vi "pane.vi"() -> ()   [LabVIEW 2015]
uses:
  <vilib>/Utility/miscctls.llb/LVPointTypeDef.ctl
panel:
  in  "Home":bool
  in  "User":bool
  in  "Devices":bool
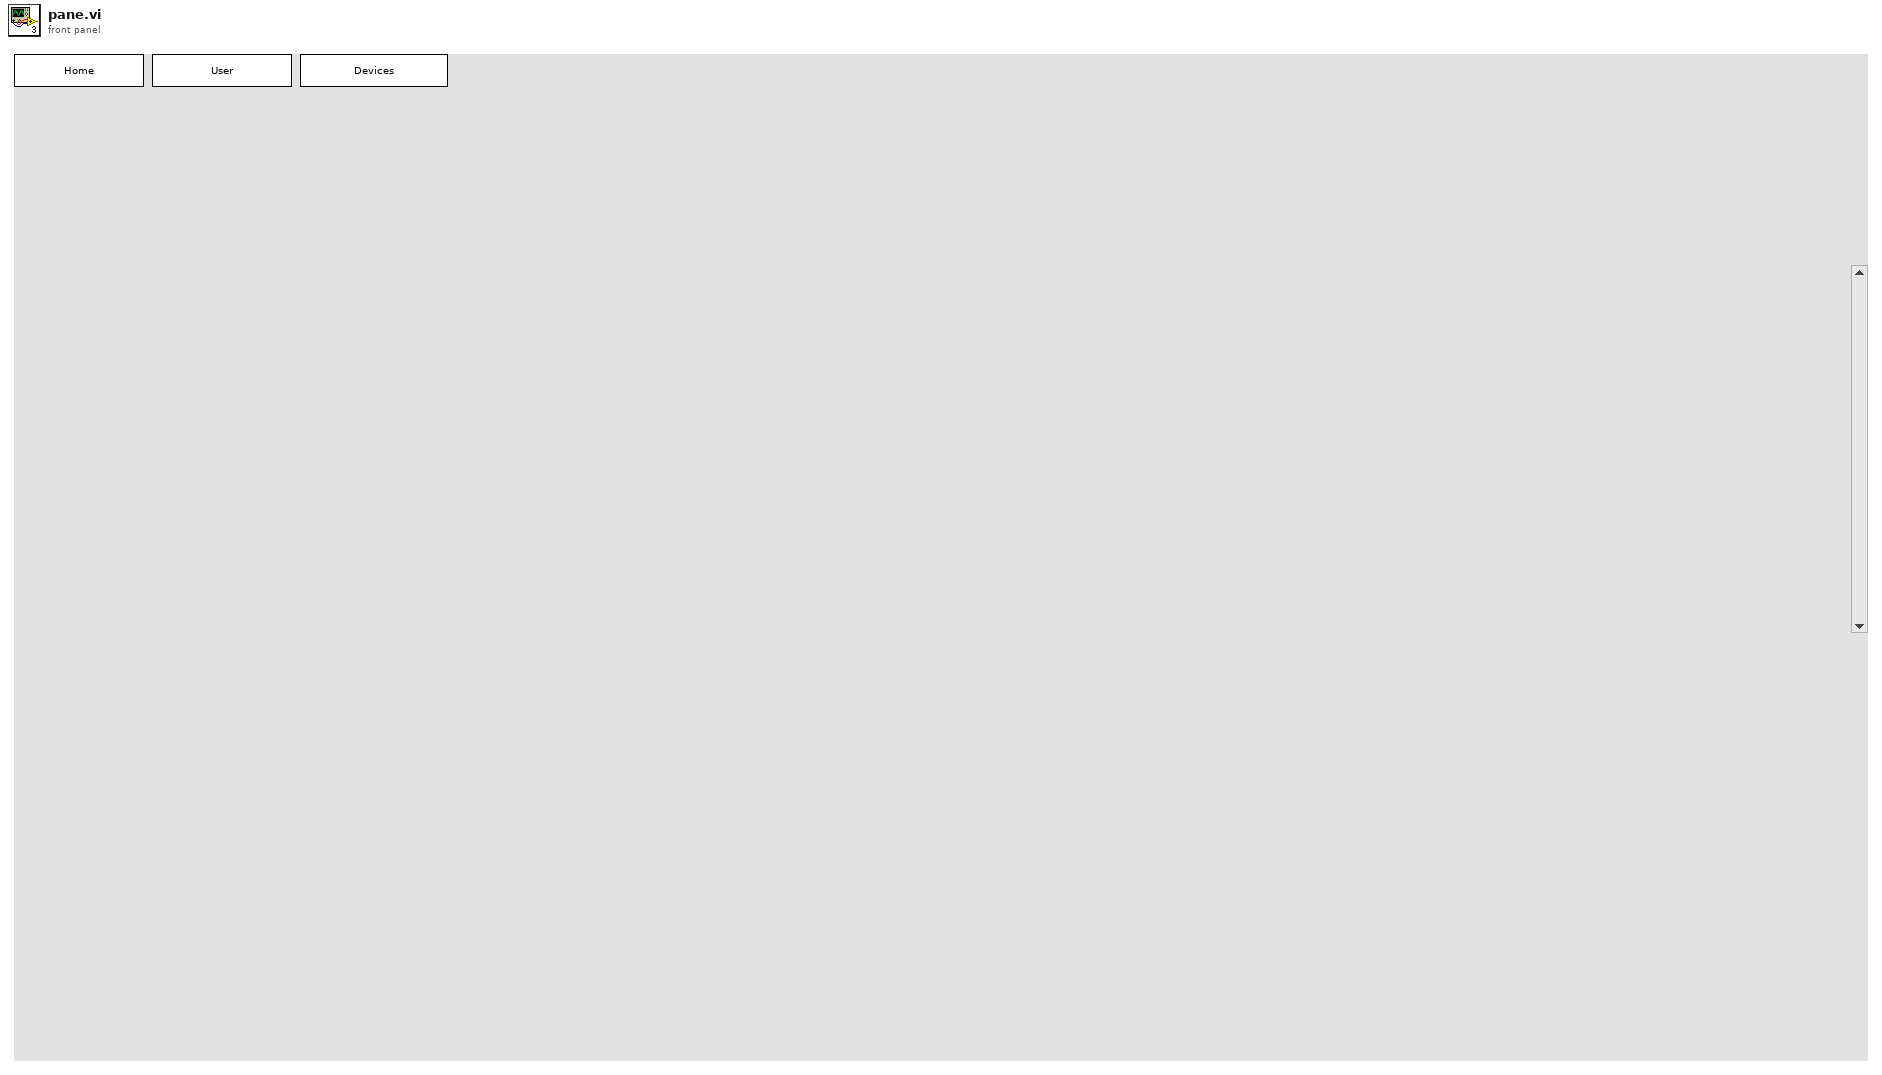
[diagram p1: front panel]
types:
  T1 = typedef "LVPointTypeDef.ctl" = cluster{"Horizontal":i16, "Vertical":i16}
  T2 = enum32{"invalid app kind", "Development System", "Run Time System", "Student Edition", "Embedded LabVIEW", "Evaluation", "Custom"}
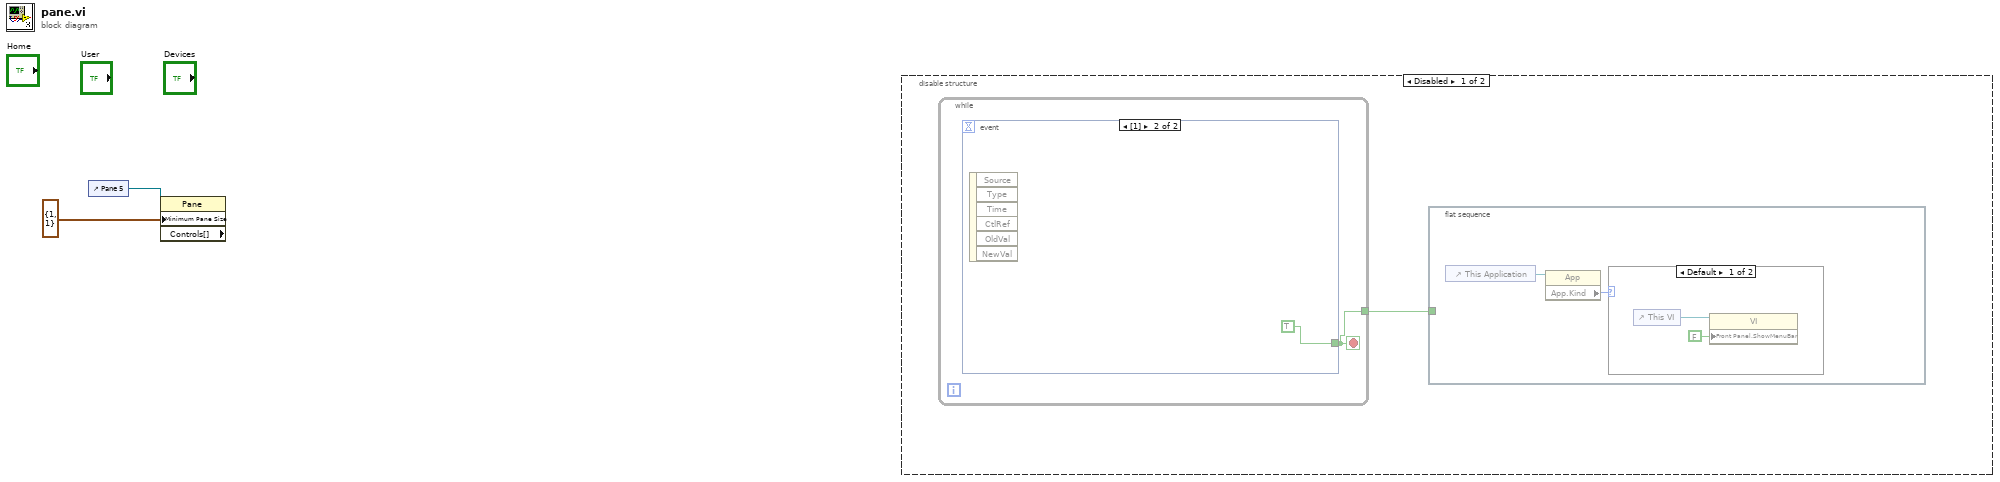
[diagram p0: block diagram]
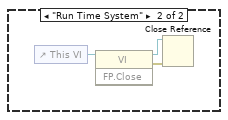
[diagram p2: hidden frame]
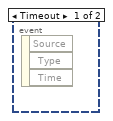
[diagram p3: hidden frame]
diagram:
  n1 = control-ref of="Pane 5"() -> (w2:refnum<vi>)
  n2 = property class="Pane" props=["Minimum Pane Size", "Controls[]"](reference=w2, "Minimum Pane Size"=T1 {"Horizontal"=1, "Vertical"=1}) -> ()  [unwired: 1 in, 3 out]
  n3 = disable-structure shown="Disabled" {
    frame Disabled {
      n4 = while {
        tunnel: [w11] -> w3
        stop <- w11 stop-if-true
        n5 = event shown="[1]" {
          selector: _ -> [_ _]
          dyn-events: _ -> [_ _]
          timeout: _ -> [_ _]
          tunnel: [_ TRUE] -> w11
          event Timeout {
            n6 = event-data() -> ()  [unwired: 1 in, 3 out]
          }
          event #1 (no event record) {
            n7 = event-data() -> ()  [unwired: 1 in, 6 out]
          }
        }
      }
      n8 = flat-sequence {
        tunnel: w3 -> [_]
        frame #0 {
          n9 = control-ref of="This Application"() -> (w5:refnum<vi>)
          n10 = property class="App"(reference=w5) -> ("App.Kind"=w4:T2)  [unwired: 1 in, 2 out]
          n11 = case shown="Default" w4 {
            frame Default {
              n12 = control-ref of="This VI"() -> (w7:refnum<vi>)
              n13 = property class="VI"(reference=w7, "Front Panel.ShowMenuBar"=FALSE ("Front Panel Window:Show Menu Bar")) -> ()  [unwired: 1 in, 2 out]
            }
            frame "Run Time System" {
              n14 = control-ref of="This VI"() -> (w10:refnum<vi>)
              n15 = invoke class="VI" method="FP.Close"(reference=w10) -> (reference out=w8:refnum<vi>, error out=w9:errorcluster)  [unwired: 2 in, 1 out]
              n16 = Close Reference(reference=w8, error in (no error)=w9) -> ()  [unwired: 1 out]
            }
          }
        }
      }
    }
    frame Enabled {
    }
  }
